vi "Default Instrument Setup.vi"(8 "error in (no error)":errorcluster, 11 "VISA resource name":refnum<visa-resource-name>) -> (0 "error out":errorcluster, 3 "VISA resource name out":refnum<visa-resource-name>)   [LabVIEW 2020, in "BK Precision 911X Series.lvlib"]
doc: "This Utility VI sends a default command string to the instrument whenever a new VISA session is opened, or the instrument is reset. Use this VI as a subVI for the Initialize and Reset VIs. Altering this VI could cause these two VIs to operate incorrectly."
uses:
  BK Precision 911X Series.lvlib
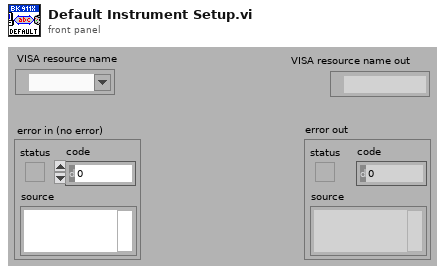
[diagram p1: front panel]
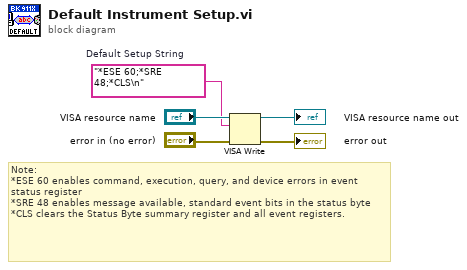
[diagram p0: block diagram]
diagram:
  w1 = "*ESE 60;*SRE 48;*CLS\n"  # Default Setup String
  # "Note:\n*ESE 60 enables command, execution, query, and device errors in event status register\n*SRE 48 enables message available, standard event bits in the status byte\n*CLS clears the Status Byte summary register and all event registers."
  n1 = VISA Write(VISA resource name="VISA resource name", write buffer=w1, error in (no error)="error in (no error)") -> (VISA resource name out=→"VISA resource name out":refnum<visa-resource-name>, error out=→"error out":errorcluster)  [unwired: 1 out]
